vi "Perform Audio Measurements.vi"(0 "Measurement Configuration":T1={"Band start"=20.0, "Band stop"=20000.0, "Weighting filter"="", "Amplitude"=1.0, "Frequency"=1000.0, "Full scale range"=3.16, "Analog source resource name"="", "Protocol capture resource name"="", "Channel name"="0L", "Data line"=0, "Sample rate"=12288000.0, "Measurement duration"=19200.0, "Channel"=0, "Frame sync edge for channel 0"=0, "Channel count per frame"=2, "Channel length"=32, "Bit depth"=24, "Channel 0 offset"=1, "Endianness"=0, "Data justification"=0, "Frame length"=64, "Frame sync pulse width"=32, "Bit clock edge sync"=1} {"Data line" format="%#.0f"}, 1 "I2S waveforms":waveform(dbl)[](array[waveform]), 3 "error in":errorcluster) -> (7 "Measurement Results":T2, 10 "error out":errorcluster)   [LabVIEW 2021, in "AC_Audio ADC.lvlib"]
uses:
  AC_Audio ADC.lvlib
  <vilib>/addons/_NISVFA/_Shared subVIs/Controls/svc_Window.ctl
  <vilib>/addons/Sound and Vibration/svt_Single Tone Measurements/SoundVib_SingleTone.lvlib
  <vilib>/addons/Sound and Vibration/svt_Single Tone Measurements/SVT Dynamic Range (Frequency) (1 Ch).vi
  <vilib>/addons/Sound and Vibration/svt_Distortion/SoundVib_Distortion.lvlib
  <vilib>/addons/Sound and Vibration/svt_Distortion/SVT SNR without Harmonics (Frequency) (1 Ch).vi
  <vilib>/addons/Sound and Vibration/svt_Single Tone Measurements/SVT Gain (Time) (1 Ch).vi
  <vilib>/addons/Sound and Vibration/svt_Single Tone Measurements/SVT Spurious Free Dynamic Range (Frequency) (1 Ch).vi
  <vilib>/addons/Sound and Vibration/svt_Weighting/SoundVib_ABCWeighting.lvlib
  Measurement Results.ctl
  <vilib>/addons/_NISVFA/_Spectrum Processing/SVFA Unit Conversion (Complex) (1 Ch).vi
  shared/audio adc shared.lvlib
  <vilib>/addons/Sound and Vibration/svt_Weighting/SVT Weighting Filter (N Ch).vi
  <vilib>/addons/_NISVFA/_Shared subVIs/Common/SVL Set dB Reference (N Ch - 1 Ref).vi
  <vilib>/addons/Sound and Vibration/svt_Level/SVL AC & DC Level (Time) (N Ch).vi
  Measurement Configuration.ctl
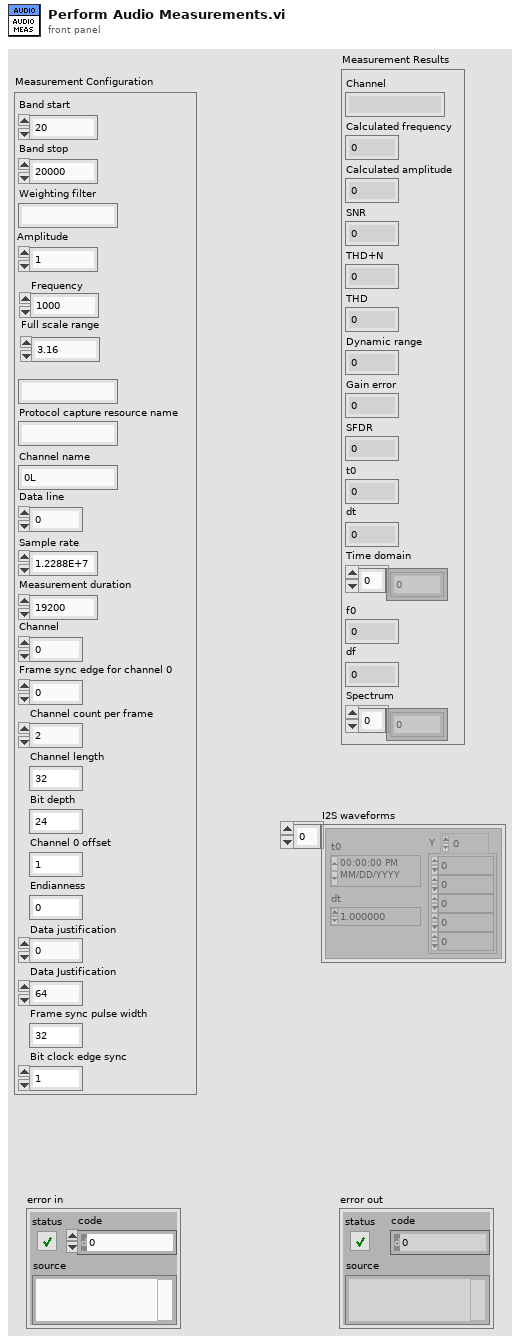
[diagram p1: front panel]
types:
  T1 = typedef "AC_Audio ADC.lvlib/Measurement Configuration.ctl" = cluster{"Band start":dbl, "Band stop":dbl, "Weighting filter":string, "Amplitude":dbl, "Frequency":dbl, "Full scale range":dbl, "Analog source resource name":string, "Protocol capture resource name":string, "Channel name":string, "Data line":u16, "Sample rate":dbl, "Measurement duration":dbl, "Channel":u32, "Frame sync edge for channel 0":u32, "Channel count per frame":u32, "Channel length":u32, "Bit depth":u32, "Channel 0 offset":u32, "Endianness":u32, "Data justification":u32, "Frame length":u32, "Frame sync pulse width":u32, "Bit clock edge sync":u32}
  T2 = typedef "AC_Audio ADC.lvlib/Measurement Results.ctl" = cluster{"Channel":string, "Calculated frequency":dbl, "Calculated amplitude":dbl, "SNR":dbl, "THD+N":dbl, "THD":dbl, "Dynamic range":dbl, "Gain error":dbl, "SFDR":dbl, "t0":dbl, "dt":dbl, "Time domain":dbl[], "f0":dbl, "df":dbl, "Spectrum":dbl[]}
  T3 = enum16{"no change", "spectrum", "spectral density"}
  T4 = cluster{"linear/dB":enum16{"no change", "linear", "dB"}, "dB reference (0: no change)":dbl, "power/magnitude":enum16{"no change", "power", "magnitude"}, "view":enum16{"no change", "rms", "peak", "peak-peak"}}
  T5 = cluster{"start frequency":dbl, "stop frequency":dbl}
  T6 = cluster{"gain units":enum16{"dB", "linear ratio"}, "detected fundamental amplitude units":enum16{"EU rms", "EU peak", "EU peak-peak"}}
  T7 = typedef "svc_Window.ctl" = u32
  T8 = cluster{"SNR units":enum16{"dB", "linear ratio", "%"}, "detected fundamental amplitude units":enum16{"EU rms", "EU peak", "EU peak-peak"}}
  T9 = typedef "svc_Spectrum Info.ctl" = cluster{"channel name":string, "description":string, "x-axis units":T10, "spectral info":cluster{"spectrum type":T11, "linear/dB":enum16{"linear", "dB"}, "window":u16, "window size":i32, "FFT size":i32}, "engineering units":T12, "custom label":string, "dB reference [EU]":dbl, "peak units":enum16{"rms", "peak", "peak-peak"}, "weighting filter":T13, "spectral density?":bool, "unit label":string, "spectrum skewed?":bool, "complimentary spectrum units":T14}
  T10 = typedef "svc_X-Axis Units.ctl" = u16
  T11 = typedef "svc_Spectrum Type.ctl" = enum16{"FFT Spectrum [complex]", "Amplitude [Magnitude]", "Power [Magnitude^2]", "Cross Spectrum [complex]", "Frequency Response [Complex]"}
  T12 = typedef "svc_Engineering Units Text Ring.ctl" = u16
  T13 = typedef "svc_Weighting Filter Text Ring.ctl" = u16
  T14 = typedef "svc_Complimentary Spectrum Units.ctl" = enum16{"none", "radians", "degrees", "cycles", "imaginary"}
  T15 = cluster{"complex spectrum response":cluster{"f0":dbl, "df":dbl, "complex spectrum":cdb[]}, "spectrum info":T9}
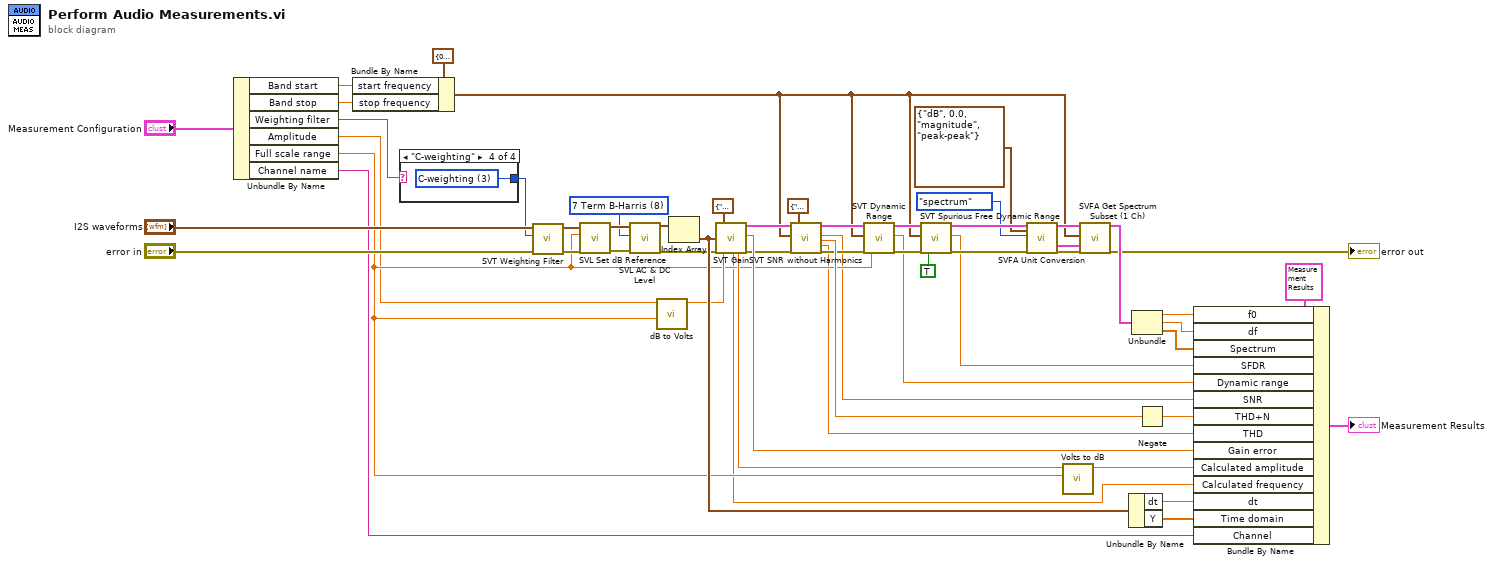
[diagram p0: block diagram]
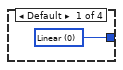
[diagram p2: hidden frame]
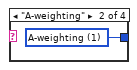
[diagram p3: hidden frame]
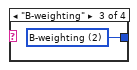
[diagram p4: hidden frame]
diagram:
  w32 = T7 8 items=["None"=0, "Hanning"=1, "Hamming"=2, "Blackman-Harris"=3, "Exact Blackman"=4, "Blackman"=5, "Flat Top"=6, "4 Term B-Harris "=7, "7 Term B-Harris"=8, "Low Sidelobe"=9, "Force"=64, "Exponential"=65, "Blackman Nuttall"=11, "Triangle"=30, "Bartlett-Hanning"=31, "Bohman"=32, "Parzen"=33, "Welch"=34, "Kaiser"=60, "Dolph-Chebyshev"=61, "Gaussian"=62] ("window")
  n1 = Unbundle By Name("Measurement Configuration") -> ("Band start"=w49:dbl, "Band stop"=w50:dbl, "Weighting filter"=w12:string, "Amplitude"=w9:dbl, "Full scale range"=w10:dbl, "Channel name"=w11:string)
  n2 = Bundle By Name(cluster=T5 {"start frequency"=0.0, "stop frequency"=0.0} ("frequency range"), "start frequency"=w49, "stop frequency"=w50) -> (w18:T5)
  n3 = case shown="\"C-weighting\"" w12 {
    tunnel: [w57 w58 w59 w60] -> w8
    frame Default {
      w57 = u16 0 items=["Linear", "A-weighting", "B-weighting", "C-weighting"] ("weighting")
    }
    frame "A-weighting" {
      w58 = u16 1 items=["Linear", "A-weighting", "B-weighting", "C-weighting"] ("weighting")
    }
    frame "B-weighting" {
      w59 = u16 2 items=["Linear", "A-weighting", "B-weighting", "C-weighting"] ("weighting")
    }
    frame "C-weighting" {
      w60 = u16 3 items=["Linear", "A-weighting", "B-weighting", "C-weighting"] ("weighting")
    }
  }
  n4 = call-poly <vilib>:"SVT Weighting Filter.vi"("error in (no error)"="error in", "weighting"=w8, "scaled signals [EU]"="I2S waveforms") -> ("error out"=w46:errorcluster, "weighted signals [EU]"=w45:waveform(dbl)[])  [unwired: 6 in]
  n5 = call-poly <vilib>:"SVL Set dB Reference.vi"("error in (no error)"=w46, "dB reference [EU]"=w10, "scaled signals in [EU]"=w45) -> ("error out"=w33:errorcluster, "scaled signals out [EU]"=w35:waveform(dbl)[])  [unwired: 7 in]
  n6 = call-poly <vilib>:"SVL AC & DC Level.vi"("scaled signals in [EU]"=w35, "window"=w32, "error in (no error)"=w33) -> ("AC signals [EU]"=w34:waveform(dbl)[], "error out"=w41:errorcluster)  [unwired: 11 in, 4 out]
  n7 = call "dB to Volts.vi"("Full scale range"=w10, "Voltage(dB)"=w9) -> ("Voltage(volts)"=w21:dbl)  [unwired: 9 in]
  n8 = Index Array(array=w34) -> (element=w53:waveform(dbl))  [unwired: 1 in]
  n9 = call-poly <vilib>:"SVT Gain.vi"("scaled signal [EU]"=w53, "error in (no error)"=w41, "desired units"=T6 {"gain units"=enum."dB", "detected fundamental amplitude units"=enum."EU peak"}, "amplitude [EU peak]"=w21) -> ("detected fundamental\nfrequency [Hz]"=w1:dbl, "detected fundamental\namplitude"=w20:dbl, "complex spectrum"=w29:T15, "gain"=w52:dbl, "error out"=w31:errorcluster)  [unwired: 10 in, 1 out]
  n10 = call-poly <vilib>:"SVT SNR without Harmonics.vi"("complex spectrum"=w29, "frequency range"=w18, "error in (no error)"=w31, "desired units"=T8 {"SNR units"=enum."dB", "detected fundamental amplitude units"=enum."EU rms"}) -> ("complex spectrum"=w37:T15, "SNR (without harmonics)"=w5:dbl, "SINAD"=w38:dbl, "THD"=w3:dbl, "error out"=w36:errorcluster)  [unwired: 8 in, 3 out]
  n11 = call-poly <vilib>:"SVT Dynamic Range.vi"("complex spectrum"=w37, "frequency range"=w18, "error in (no error)"=w36, "full scale amplitude [EU peak]"=w10) -> ("dup complex spectrum"=w42:T15, "dynamic range"=w6:dbl, "error out"=w43:errorcluster)  [unwired: 10 in, 3 out]
  n12 = call-poly <vilib>:"SVT Spurious Free Dynamic Range.vi"("complex spectrum"=w42, "frequency range"=w18, "error in (no error)"=w43, "exclude harmonics"=TRUE) -> ("complex spectrum"=w27:T15, "spurious free dynamic range"=w7:dbl, "error out"=w28:errorcluster)  [unwired: 8 in, 5 out]
  n13 = call-poly <vilib>:"SVFA Unit Conversion.vi"("complex spectrum"=w27, "desired scaling"=T4 {"linear/dB"=enum."dB", "dB reference (0: no change)"=0.0, "power/magnitude"=enum."magnitude", "view"=enum."peak-peak"}, "spectral density desired"=T3."spectrum", "error in (no error)"=w28) -> ("converted spectrum"=w19:cluster{"x0":dbl, "dx":dbl, "magnitude":dbl[]}, "spectrum info out"=w15:T9, "error out"=w14:errorcluster)  [unwired: 10 in, 3 out]
  n14 = call "Volts to dB.vi"("Full scale range"=w10, "Voltage(V)"=w20) -> ("Voltage(dB)"=w2:dbl)  [unwired: 9 in]
  n15 = call <vilib>:"SVFA Get Spectrum Subset (1 Ch).vi"("spectrum"=w19, "range"=w18, "spectrum info"=w15, "error in (no error)"=w14) -> ("spectrum subset"=w17:cluster{"x0":dbl, "dx":dbl, "magnitude":dbl[]}, "error out"=→"error out":errorcluster)  [unwired: 10 in, 4 out]
  n16 = Unbundle By Name ("Get Waveform Components")(w53) -> ("dt"=w54:dbl, "Y"=w55:dbl[])
  n17 = Unbundle(w17) -> ("x0"=w24:dbl, "dx"=w23:dbl, "magnitude"=w22:dbl[])
  n18 = Negate(x=w38) -> (-x=w4:dbl)
  n19 = Bundle By Name(cluster=T2 {"Channel"="", "Calculated frequency"=0.0, "Calculated amplitude"=0.0, "SNR"=0.0, "THD+N"=0.0, "THD"=0.0, "Dynamic range"=0.0, "Gain error"=0.0, "SFDR"=0.0, "t0"=0.0, "dt"=0.0, "Time domain"=[], "f0"=0.0, "df"=0.0, "Spectrum"=[]} ("Measurement Results"), "f0"=w24, "df"=w23, "Spectrum"=w22, "SFDR"=w7, "Dynamic range"=w6, "SNR"=w5, "THD+N"=w4, "THD"=w3, "Gain error"=w52, "Calculated amplitude"=w2, "Calculated frequency"=w1, "dt"=w54, "Time domain"=w55, "Channel"=w11) -> (→"Measurement Results":T2)
